vi "Teleop.vi"(10 "Match Info":T2={"Autonomous Elapsed Seconds"=0.0, "TeleOp Elapsed Seconds"=43.396, "Disabled Elapsed Seconds"=3.878, "Visited Autonomous"=FALSE, "Visited TeleOp"=TRUE, "Visited Disabled"=TRUE, "Autonomous Settings"={"Autonomous Style"=enum."Independent", "VI Refnum"=refnum}}, 11 "Call Context":T3=enum."Execute") -> ()   [LabVIEW 2017]
doc: "This VI is called for each TeleOp packet received from the DS where the robot is not disabled. It is often used to read from the joysticks and update I/O or to update setpoints for timed control loops. It should complete and return within 20 milliseconds or it may miss DS packets."
uses:
  <vilib>/Rock Robotics/WPI/DriverStation/WPI_DriverStationDerivedRobotMode.ctl
  <vilib>/Rock Robotics/WPI/DriverStation/WPI_DriverStationMatch Info.ctl
  <vilib>/Rock Robotics/WPI/Solenoid/WPI_SolenoidValue.ctl
  Public/Documents/Cross The Road Electronics/Phoenix-LabVIEW/Motor Controller/Controls/CTRE_Phoenix_MotorControl_ControlMode.ctl
  <vilib>/Rock Robotics/WPI/Utilities/WPI_GetSetVariantRefNum.vi
  <vilib>/Rock Robotics/Network Tables/NT Write Boolean Array.vi
  <vilib>/Rock Robotics/Network Tables/NT Write Numeric Array.vi
  <vilib>/Rock Robotics/Network Tables/NT Read Boolean.vi
  <vilib>/Rock Robotics/Network Tables/NT Read Number.vi
  <vilib>/addons/control/pid/pid.llb/PID (DBL).vi
  <vilib>/Rock Robotics/WPI/Solenoid/WPI_SolenoidSetEnum.vi
  Public/Documents/Cross The Road Electronics/Phoenix-LabVIEW/Motor Controller/Get/CTRE_Phoenix_MotorController_GetSelectedSensorData.vi
  FIRST-3958-Controls-Library/NavX/navX Library v2/navX Library v2.lvlib
  <vilib>/addons/control/pid/NI_PID_pid.lvlib
panel:
  out "elevator position":i32=2052
  in  "elevator PID":T1={"proportional gain (Kc)"=0.005, "integral time (Ti, min)"=0.0, "derivative time (Td, min)"=0.0} {"derivative time (Td, min)" format="%.3f"; "integral time (Ti, min)" format="%.3f"; "proportional gain (Kc)" format="%.3f"}
  in  "elevator setpoint":dbl=2050.0 format="%.2f"
  out "Scale":dbl(slide)=0.49834983498349833 scale=0.0..1.0
  out "error out 2":errorcluster
  out "error out":errorcluster
  out "Sample Slider 0":dbl(slide) scale=0.0..5.0
  out "Sample Boolean 1":bool
  out "Sample Boolean 0":bool
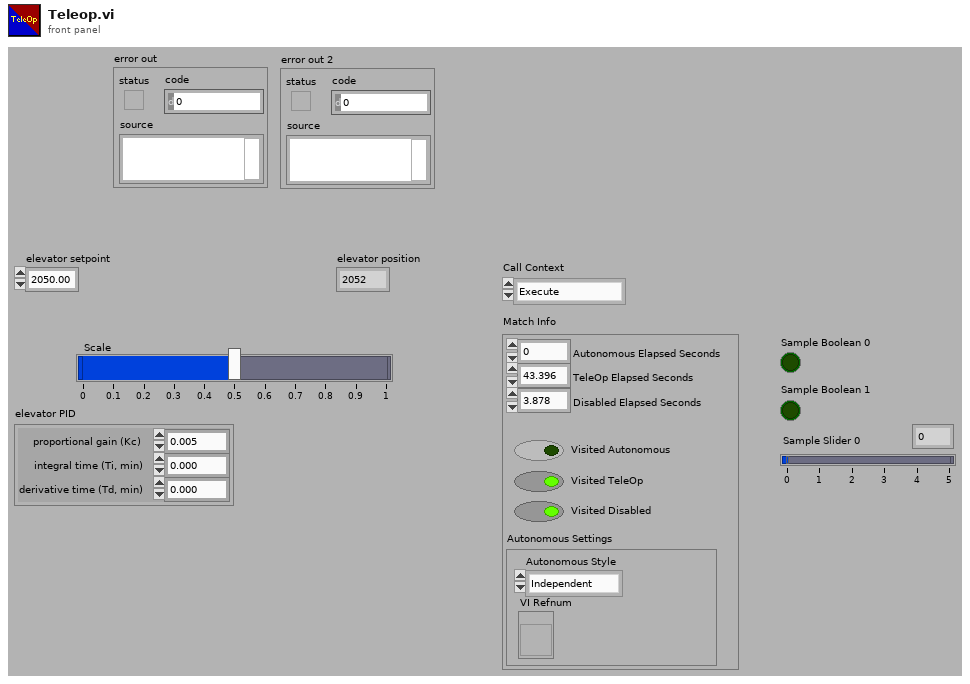
[diagram p1: front panel]
types:
  T1 = cluster{"proportional gain (Kc)":dbl, "integral time (Ti, min)":dbl, "derivative time (Td, min)":dbl}
  T2 = typedef "WPI_DriverStationMatch Info.ctl" = cluster{"Autonomous Elapsed Seconds":dbl, "TeleOp Elapsed Seconds":dbl, "Disabled Elapsed Seconds":dbl, "Visited Autonomous":bool, "Visited TeleOp":bool, "Visited Disabled":bool, "Autonomous Settings":cluster{"Autonomous Style":enum16{"Iterative", "Independent"}, "VI Refnum":refnum<vi>}}
  T3 = typedef "WPI_DriverStationDerivedRobotMode.ctl" = enum16{"Init", "Execute", "Stop"}
  T4 = typedef "CTRE_Phoenix_MotorControl_ControlMode.ctl" = u16
  T5 = typedef "WPI_SolenoidValue.ctl" = enum16{"Off", "On", "Forward", "Reverse"}
  T6 = typedef "WPI_JoystickDevRef.ctl" = cluster{"Device":T7}
  T7 = typedef "WPI_JoystickDeviceEnum.ctl" = enum16{"USB 0", "USB 1", "USB 2", "USB 3", "USB 4", "USB 5"}
  T8 = typedef "WPI_RobotDriveDevRef.ctl" = cluster{"DevStatus":errorcluster, "Motors[]":T9[], "Square Inputs":bool, "Max Output":dbl}
  T9 = typedef "WPI_MotorControlDeviceRef.ctl" = cluster{"DeviceStatus":errorcluster, "Type":T10, "PWM":cluster{"PWM Channel":T11, "DeadBand":T12}, "CAN":cluster{"Device Number":u8, "SetOutput VI Ref":variant, "GetOutput VI Ref":variant, "Enable VI Ref":variant, "Disable VI Ref":variant, "Data":variant}, "Invert":bool, "DIO PWM":cluster{"PWM \"Enable\" Channel":T11, "DIOChannel":T13, "PWM Rate":dbl}}
  T10 = typedef "WPI_MotorControlType.ctl" = enum16{"PWM", "CAN", "DIO PWM"}
  T11 = typedef "FPGA_DIOPWMChannel.ctl" = enum8{"PWM 0", "PWM 1", "PWM 2", "PWM 3", "PWM 4", "PWM 5", "PWM 6", "PWM 7", "PWM 8", "PWM 9", "PWM MXP 0", "PWM MXP 1", "PWM MXP 2", "PWM MXP 3", "PWM MXP 4", "PWM MXP 5", "PWM MXP 6", "PWM MXP 7", "PWM MXP 8", "PWM MXP 9", "Invalid"}
  T12 = typedef "WPI_PWMDeadband.ctl" = cluster{"Name":string, "maxPositivePwm":i32, "minPositivePwm":i32, "centerPwm":i32, "maxNegativePwm":i32, "minNegativePwm":i32, "angularRange":u16}
  T13 = typedef "FPGA_DIOChannel.ctl" = enum8{"DIO 0", "DIO 1", "DIO 2", "DIO 3", "DIO 4", "DIO 5", "DIO 6", "DIO 7", "DIO 8", "DIO 9", "DIO MXP 0", "DIO MXP 1", "DIO MXP 2", "DIO MXP 3", "DIO MXP 4", "DIO MXP 5", "DIO MXP 6", "DIO MXP 7", "DIO MXP 8", "DIO MXP 9", "DIO MXP 10", "DIO MXP 11", "DIO MXP 12", "DIO MXP 13", "DIO MXP 14", "DIO MXP 15", "SPI Port CS1", "SPI Port CS2", "SPI Port CS3", "SPI Port MISO", "SPI Port MOSI", "Invalid"}
  T14 = typedef "WPI_ServoDeviceRef.ctl" = cluster{"DeviceStatus":errorcluster, "PWM Channel":T11, "DeadBand":T12}
  T15 = typedef "navX Library v2.lvlib/Z900_navX_DeviceTypeDef.ctl" = cluster{"Interface":cluster{"Protocol":T16, "Update Rate (4Hz-100Hz)":u8, "navX Open TypeDef":variant}, "Notify Packet":refnum<notifier>, "Loop VI Refnum":refnum<vi>, "Ready to Close Occurrence Refnum":refnum<k4>}
  T16 = typedef "navX Library v2.lvlib/Z900_navX_ProtocolTypeDef.ctl" = enum16{"SERIAL", "I2C", "SPI"}
  T17 = cluster{"Yaw":dbl, "Roll":dbl, "Pitch":dbl, "Heading":dbl, "Fused Heading":dbl}
  T18 = typedef "WPI_SolenoidDevRef.ctl" = cluster{"DevStatus":errorcluster, "Pneumatics Control Module":u8, "Forward Solenoid Channel":T19, "Reverse Solenoid Channel":T19}
  T19 = typedef "WPI_SolenoidChannel.ctl" = enum8{"Solenoid 0", "Solenoid 1", "Solenoid 2", "Solenoid 3", "Solenoid 4", "Solenoid 5", "Solenoid 6", "Solenoid 7", "Invalid"}
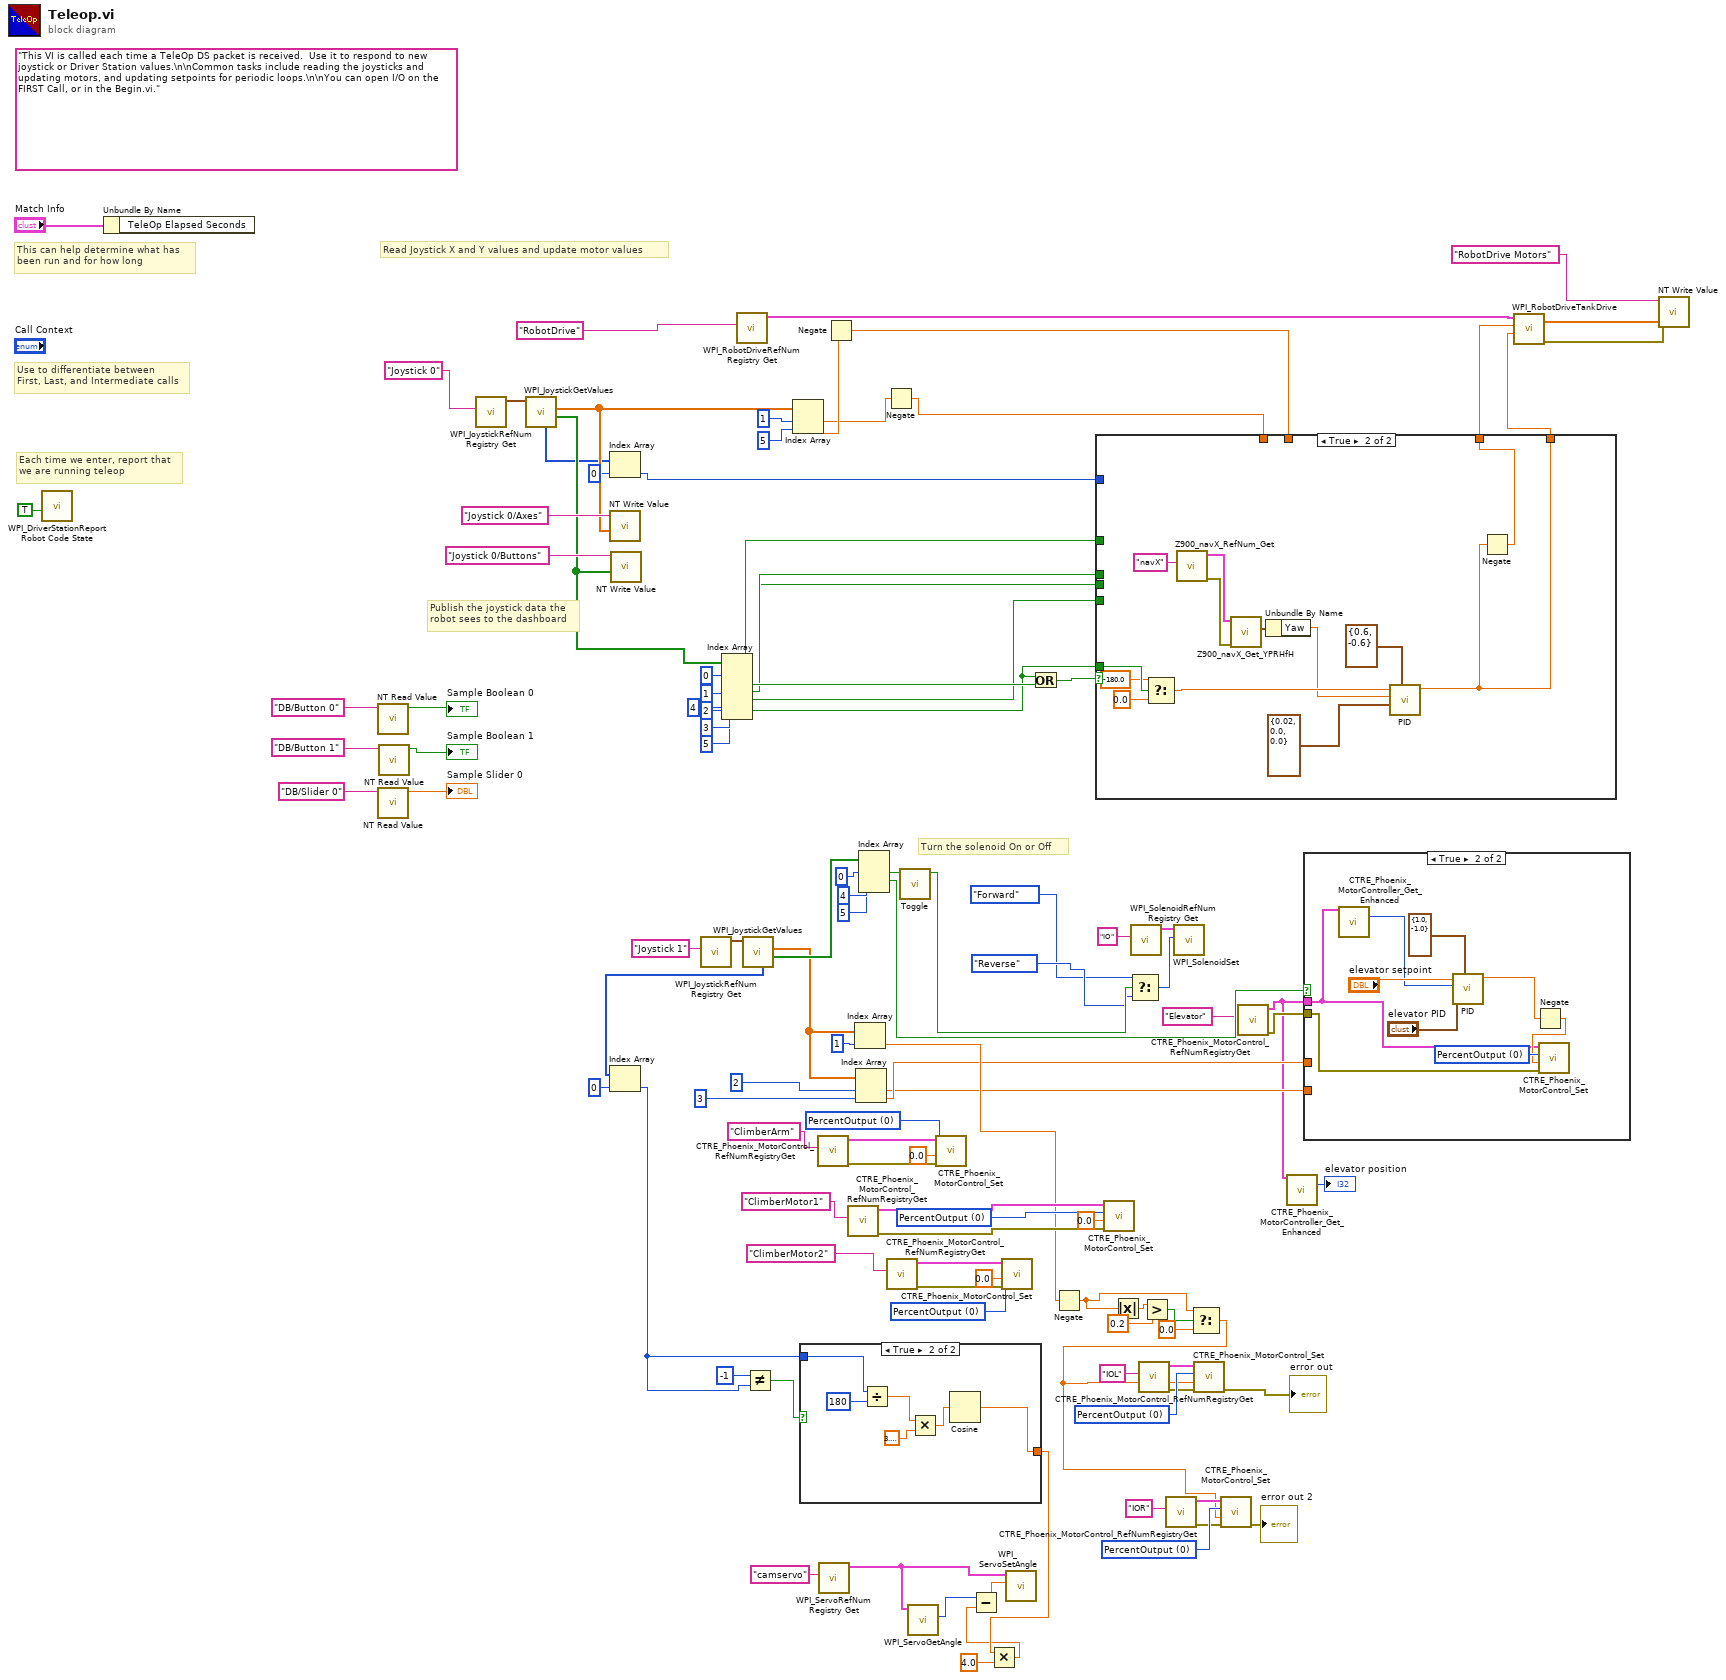
[diagram p0: block diagram]
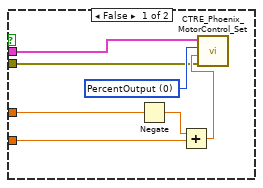
[diagram p2: hidden frame]
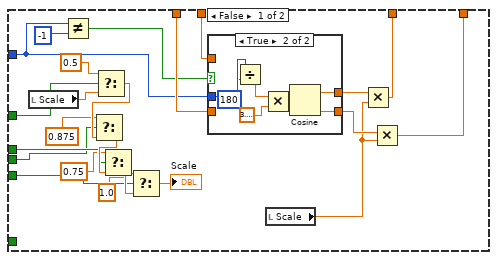
[diagram p3: hidden frame]
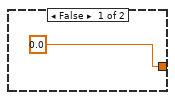
[diagram p5: hidden frame]
diagram:
  w52 = T4 0 items=["PercentOutput"=0, "Position"=1, "Velocity"=2, "Current"=3, "Follower"=5, "MotionProfile"=6, "MotionMagic"=7, "MotionMagicArc"=8, "MotionProfileArc"=10, "Disabled"=15] ("Control Mode")
  w53 = T4 0 items=["PercentOutput"=0, "Position"=1, "Velocity"=2, "Current"=3, "Follower"=5, "MotionProfile"=6, "MotionMagic"=7, "MotionMagicArc"=8, "MotionProfileArc"=10, "Disabled"=15] ("Control Mode")
  w54 = T4 0 items=["PercentOutput"=0, "Position"=1, "Velocity"=2, "Current"=3, "Follower"=5, "MotionProfile"=6, "MotionMagic"=7, "MotionMagicArc"=8, "MotionProfileArc"=10, "Disabled"=15] ("Control Mode")
  w84 = T4 0 items=["PercentOutput"=0, "Position"=1, "Velocity"=2, "Current"=3, "Follower"=5, "MotionProfile"=6, "MotionMagic"=7, "MotionMagicArc"=8, "MotionProfileArc"=10, "Disabled"=15] ("Control Mode")
  w87 = T4 0 items=["PercentOutput"=0, "Position"=1, "Velocity"=2, "Current"=3, "Follower"=5, "MotionProfile"=6, "MotionMagic"=7, "MotionMagicArc"=8, "MotionProfileArc"=10, "Disabled"=15] ("Control Mode")
  (unwired) "This VI is called each time a TeleOp DS packet is received.  Use it to respond to new joystick or Driver Station values.\n\nCommon tasks include reading the joysticks and updating motors, and updating setpoints for periodic loops.\n\nYou can open I/O on the FIRST Call, or in the Begin.vi."
  # "Turn the solenoid On or Off"
  # "Publish the joystick data the\nrobot sees to the dashboard"
  # "Each time we enter, report that\nwe are running teleop"
  # "Use to differentiate between\nFirst, Last, and Intermediate calls"
  # "This can help determine what has\nbeen run and for how long"
  # "Read Joystick X and Y values and update motor values"
  n1 = call <vilib>:"WPI_DriverStationReport Robot Code State.vi"("TeleOp"=TRUE ("Autonomous")) -> ()  [unwired: 10 in, 1 out]
  n2 = Unbundle By Name("Match Info") -> ()  [unwired: 1 out]
  n3 = call-poly <vilib>:"NT Read Value.vi"("Name"="DB/Button 0" ("refnum name")) -> ("Boolean"=→"Sample Boolean 0":bool)  [unwired: 9 in, 1 out]
  n4 = call-poly <vilib>:"NT Read Value.vi"("Name"="DB/Slider 0" ("refnum name")) -> ("Numeric"=→"Sample Slider 0":dbl)  [unwired: 9 in, 1 out]
  n5 = call-poly <vilib>:"NT Read Value.vi"("Name"="DB/Button 1" ("refnum name")) -> ("Boolean"=→"Sample Boolean 1":bool)  [unwired: 9 in, 1 out]
  n6 = call <vilib>:"WPI_JoystickRefNum Registry Get.vi"("refnum name"="Joystick 0") -> ("JoystickDevRef"=w109:T6)  [unwired: 1 in, 9 out]
  n7 = call <vilib>:"WPI_JoystickGetValues.vi"("JoystickDevRef"=w109) -> ("Buttons"=w67:bool[], "Axes"=w105:dbl[], "POVs"=w42:i16[])  [unwired: 6 in, 2 out]
  n8 = Index Array(array=w42, index=0) -> (element=w31:i16)
  n9 = call-poly <vilib>:"NT Write Value.vi"("Numeric Array"=w105, "Name"="Joystick 0/Axes") -> ()  [unwired: 9 in, 1 out]
  n10 = call-poly <vilib>:"NT Write Value.vi"("Boolean Array"=w67, "Name"="Joystick 0/Buttons") -> ()  [unwired: 9 in, 1 out]
  n11 = call <vilib>:"WPI_JoystickRefNum Registry Get.vi"("refnum name"="Joystick 1") -> ("JoystickDevRef"=w89:T6)  [unwired: 1 in, 9 out]
  n12 = Index Array(array=w67, index #1=0 ("index"), index #2=1 ("index"), index #3=2 ("index"), index #4=3 ("index"), index #5=4 ("index"), index #6=5 ("index")) -> (element #1=w32:bool, element #2=w33:bool, element #3=w34:bool, element #4=w35:bool, element #5=w36:bool, element #6=w38:bool)
  n13 = call <vilib>:"WPI_RobotDriveRefNum Registry Get.vi"("refnum name"="RobotDrive") -> ("RobotDriveDevRef"=w71:T8)  [unwired: 9 in, 1 out]
  n14 = call <vilib>:"WPI_JoystickGetValues.vi"("JoystickDevRef"=w89) -> ("Buttons"=w81:bool[], "Axes"=w66:dbl[], "POVs"=w51:i16[])  [unwired: 6 in, 2 out]
  n15 = Index Array(array=w51, index=0) -> (element=w47:i16)
  n16 = Not Equal?(x=i16 -1, y=w47) -> (x != y?=w48:bool)
  n17 = Index Array(array=w105, index #1=1 ("index"), index #2=5 ("index")) -> (element #1=w94:dbl, element #2=w95:dbl)
  n18 = case shown="True" w48 {
    tunnel: w47 -> [_ w117]
    tunnel: [0.0 w118] -> w11
    frame False {
    }
    frame True {
      n19 = Divide(x=w117, y=i16 180) -> (x/y=w115:dbl)
      n20 = Multiply(x=w115, y=3.141592653589793) -> (x*y=w113:dbl)
      n21 = Cosine(x=w113) -> (cos(x)=w118:dbl)
    }
  }
  n22 = call "CTRE_Phoenix_MotorControl_RefNumRegistryGet.vi"("refnum name"="ClimberArm") -> ("error out"=w63:errorcluster, "PhoenixMotorControlDevRef"=w64:T9)  [unwired: 9 in]
  n23 = call <vilib>:"WPI_ServoRefNum Registry Get.vi"("refnum name"="camservo") -> ("ServoDeviceRef"=w12:T14)  [unwired: 9 in, 1 out]
  n24 = Negate(x=w95) -> (-x=w29:dbl)
  n25 = call "CTRE_Phoenix_MotorControl_RefNumRegistryGet.vi"("refnum name"="ClimberMotor1") -> ("error out"=w58:errorcluster, "PhoenixMotorControlDevRef"=w59:T9)  [unwired: 9 in]
  n26 = Index Array(array=w66, index=1) -> (element=w23:dbl)
  n27 = Index Array(array=w66, index #1=2 ("index"), index #2=3 ("index")) -> (element #1=w18:dbl, element #2=w19:dbl)
  n28 = Index Array(array=w81, index #1=0 ("index"), index #2=4 ("index"), index #3=5 ("index")) -> (element #1=w78:bool, element #2=w20:bool)  [unwired: 1 out]
  n29 = Negate(x=w94) -> (-x=w30:dbl)
  n30 = call "CTRE_Phoenix_MotorControl_RefNumRegistryGet.vi"("refnum name"="ClimberMotor2") -> ("error out"=w55:errorcluster, "PhoenixMotorControlDevRef"=w56:T9)  [unwired: 9 in]
  n31 = call "Toggle.vi"("Button Input"=w78) -> ("Toggle Output"=w79:bool)  [unwired: 9 in, 1 out]
  n32 = call <vilib>:"WPI_ServoGetAngle.vi"("ServoDeviceRef"=w12) -> ("Angle"=w8:u16)  [unwired: 7 in, 2 out]
  n33 = call "CTRE_Phoenix_MotorControl_Set.vi"("error in (no error)"=w63, "Output"=0.0, "Control Mode"=w54, "PhoenixMotorControlDevRef"=w64) -> ()  [unwired: 6 in, 2 out]
  n34 = Multiply(x=w11, y=4.0) -> (x*y=w9:dbl)
  n35 = Subtract(x=w8, y=w9) -> (x-y=w7:dbl)
  n36 = call "CTRE_Phoenix_MotorControl_Set.vi"("error in (no error)"=w55, "Output"=0.0, "Control Mode"=w52, "PhoenixMotorControlDevRef"=w56) -> ()  [unwired: 6 in, 2 out]
  n37 = call <vilib>:"WPI_ServoSetAngle.vi"("Angle"=w7, "ServoDeviceRef"=w12) -> ()  [unwired: 8 in, 2 out]
  n38 = Or(x=w36, y=w38) -> (x .or. y?=w37:bool)
  n39 = Negate(x=w23) -> (-x=w3:dbl)
  n40 = case shown="True" w37 {
    tunnel: w36 -> [_ w162]
    tunnel: w35 -> [w137 _]
    tunnel: w34 -> [w135 _]
    tunnel: w33 -> [w133 _]
    tunnel: w32 -> [w131 _]
    tunnel: w31 -> [w121 _]
    tunnel: w30 -> [w128 _]
    tunnel: w29 -> [w127 _]
    tunnel: [w125 w152] -> w28
    tunnel: [w123 w151] -> w27
    frame False {
      n41 = local read "Scale"() -> (w138:dbl)
      n42 = Not Equal?(x=w121, y=i16 -1) -> (x != y?=w120:bool)
      n43 = Select(t=0.5 ("f"), s=w131, f=w138) -> (s? t:f=w139:dbl)
      n44 = Select(t=0.875 ("f"), s=w133, f=w139) -> (s? t:f=w140:dbl)
      n45 = Select(t=0.75 ("f"), s=w135, f=w140) -> (s? t:f=w141:dbl)
      n46 = Select(t=1.0 ("f"), s=w137, f=w141) -> (s? t:f=→"Scale":dbl)
      n47 = case shown="True" w120 {
        tunnel: w121 -> [_ w148]
        tunnel: [w143 w149] -> w124
        tunnel: w128 -> [w143 _]
        tunnel: [w142 w149] -> w126
        tunnel: w127 -> [w142 _]
        frame False {
        }
        frame True {
          n48 = Divide(x=w148, y=i16 180) -> (x/y=w145:dbl)
          n49 = Multiply(x=w145, y=3.141592653589793) -> (x*y=w144:dbl)
          n50 = Cosine(x=w144) -> (cos(x)=w149:dbl)
        }
      }
      n51 = local read "Scale"() -> (w122:dbl)
      n52 = Multiply(x=w126, y=w122) -> (x*y=w125:dbl)
      n53 = Multiply(x=w124, y=w122) -> (x*y=w123:dbl)
    }
    frame True {
      n54 = Select(t=-180.0, s=w162, f=0.0) -> (s? t:f=w159:dbl)
      n55 = call "Z900_navX_RefNum_Get.vi"("refnum name"="navX") -> ("error out"=w157:errorcluster, "navX Device"=w150:T15)  [unwired: 9 in]
      n56 = call "Z900_navX_Get_YPRHfH.vi"("error in (no error)"=w157, "navX Device"=w150) -> ("YRPHfH"=w158:T17)  [unwired: 6 in, 3 out]
      n57 = Unbundle By Name(w158) -> ("Yaw"=w155:dbl)
      n58 = call-poly <vilib>:"PID.vi"("output range"=cluster{"output high":dbl, "output low":dbl} {"output high"=0.6, "output low"=-0.6}, "PID gains"=T1 {"proportional gain (Kc)"=0.02, "integral time (Ti, min)"=0.0, "derivative time (Td, min)"=0.0}, "process variable"=w155, "setpoint"=w159) -> ("output"=w151:dbl)  [unwired: 6 in, 1 out]
      n59 = Negate(x=w151) -> (-x=w152:dbl)
    }
  }
  n60 = call "CTRE_Phoenix_MotorControl_Set.vi"("error in (no error)"=w58, "Output"=0.0, "Control Mode"=w53, "PhoenixMotorControlDevRef"=w59) -> ()  [unwired: 6 in, 2 out]
  n61 = Absolute Value(x=w3) -> (abs(x)=w6:dbl)
  n62 = Select(t=WPI_SolenoidValue."Forward" ("Value"), s=w79, f=WPI_SolenoidValue."Reverse" ("Value")) -> (s? t:f=w93:T5)
  n63 = call <vilib>:"WPI_SolenoidRefNum Registry Get.vi"("refnum name"="IO") -> ("SolenoidDevRef"=w91:T18)  [unwired: 9 in, 1 out]
  n64 = call "CTRE_Phoenix_MotorControl_RefNumRegistryGet.vi"("refnum name"="IOL") -> ("error out"=w77:errorcluster, "PhoenixMotorControlDevRef"=w86:T9)  [unwired: 9 in]
  n65 = Greater?(x=w6, y=0.2) -> (0:w4:bool)
  n66 = call "CTRE_Phoenix_MotorControl_RefNumRegistryGet.vi"("refnum name"="IOR") -> ("error out"=w76:errorcluster, "PhoenixMotorControlDevRef"=w83:T9)  [unwired: 9 in]
  n67 = call-poly <vilib>:"WPI_SolenoidSet.vi"("Value"=w93, "SolenoidDevRef"=w91) -> ()  [unwired: 1 in, 9 out]
  n68 = Select(t=w3, s=w4, f=0.0) -> (s? t:f=w1:dbl)
  n69 = call "CTRE_Phoenix_MotorControl_Set.vi"("error in (no error)"=w77, "Output"=w1, "Control Mode"=w87, "PhoenixMotorControlDevRef"=w86) -> ("error out"=→"error out":errorcluster)  [unwired: 6 in, 1 out]
  n70 = call "CTRE_Phoenix_MotorControl_Set.vi"("error in (no error)"=w76, "Output"=w1, "Control Mode"=w84, "PhoenixMotorControlDevRef"=w83) -> ("error out"=→"error out 2":errorcluster)  [unwired: 6 in, 1 out]
  n71 = call "CTRE_Phoenix_MotorControl_RefNumRegistryGet.vi"("refnum name"="Elevator") -> ("error out"=w16:errorcluster, "PhoenixMotorControlDevRef"=w15:T9)  [unwired: 9 in]
  n72 = call-poly "CTRE_Phoenix_MotorController_Get_Enhanced.vi"("PhoenixMotorControlDevRef"=w15) -> ("Position (Raw Sensor Units)"=→"elevator position":i32)  [unwired: 11 in, 3 out]
  n73 = case shown="True" w20 {
    tunnel: w19 -> [w167 _]
    tunnel: w18 -> [w166 _]
    tunnel: w16 -> [w164 w176]
    tunnel: w15 -> [w163 w171]
    frame False {
      w165 = T4 0 items=["PercentOutput"=0, "Position"=1, "Velocity"=2, "Current"=3, "Follower"=5, "MotionProfile"=6, "MotionMagic"=7, "MotionMagicArc"=8, "MotionProfileArc"=10, "Disabled"=15] ("Control Mode")
      n74 = Negate(x=w167) -> (-x=w169:dbl)
      n75 = Add(x=w169, y=w166) -> (x+y=w168:dbl)
      n76 = call "CTRE_Phoenix_MotorControl_Set.vi"("error in (no error)"=w164, "Output"=w168, "Control Mode"=w165, "PhoenixMotorControlDevRef"=w163) -> ()  [unwired: 6 in, 2 out]
    }
    frame True {
      w175 = T4 0 items=["PercentOutput"=0, "Position"=1, "Velocity"=2, "Current"=3, "Follower"=5, "MotionProfile"=6, "MotionMagic"=7, "MotionMagicArc"=8, "MotionProfileArc"=10, "Disabled"=15] ("Control Mode")
      n77 = call-poly "CTRE_Phoenix_MotorController_Get_Enhanced.vi"("PhoenixMotorControlDevRef"=w171) -> ("Position (Raw Sensor Units)"=w170:i32)  [unwired: 11 in, 3 out]
      n78 = call-poly <vilib>:"PID.vi"("output range"=cluster{"output high":dbl, "output low":dbl} {"output high"=1.0, "output low"=-1.0}, "PID gains"="elevator PID", "process variable"=w170, "setpoint"="elevator setpoint") -> ("output"=w173:dbl)  [unwired: 6 in, 1 out]
      n79 = Negate(x=w173) -> (-x=w172:dbl)
      n80 = call "CTRE_Phoenix_MotorControl_Set.vi"("error in (no error)"=w176, "Output"=w172, "Control Mode"=w175, "PhoenixMotorControlDevRef"=w171) -> ()  [unwired: 6 in, 2 out]
    }
  }
  n81 = call <vilib>:"WPI_RobotDriveTankDrive.vi"("Right axis value"=w27, "Left axis value"=w28, "RobotDriveDevRef"=w71) -> ("error out"=w69:errorcluster, "Motor Values"=w70:dbl[])  [unwired: 6 in, 1 out]
  n82 = call-poly <vilib>:"NT Write Value.vi"("error in"=w69, "Numeric Array"=w70, "Name"="RobotDrive Motors") -> ()  [unwired: 8 in, 1 out]
